vi "isDone.vi"(8 "error in (no error)":errorcluster, 11 "ChirpWave in":refnum<class "ChirpWave.lvclass">) -> (0 "error out":errorcluster, 2 "isDone?":bool=TRUE, 3 "ChirpWave out":refnum<class "ChirpWave.lvclass">)   [LabVIEW 2015, in "ChirpWave.lvclass"]
uses:
  ChirpWave.lvclass
  ChirpWave.lvclass/ChirpWave.ctl
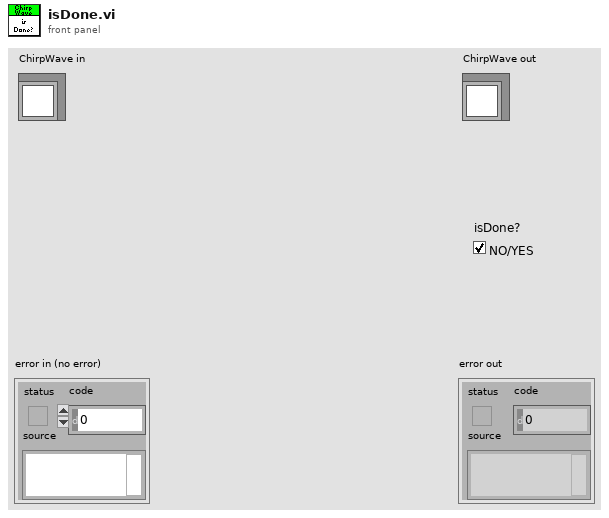
[diagram p1: front panel]
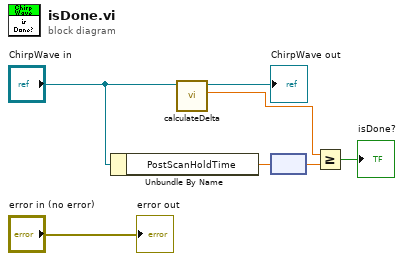
[diagram p0: block diagram]
diagram:
  n1 = Unbundle By Name("ChirpWave in") -> ("PostScanHoldTime"=w2:dbl[unit])
  n2 = call "calculateDelta.vi"("ChirpWave in"="ChirpWave in") -> ("Delta Timestamp"=w5:dbl, "ChirpWave out"=→"ChirpWave out":refnum<class "ChirpWave.lvclass">)  [unwired: 8 in, 1 out]
  n3 = node(w2) -> (w3:dbl)
  n4 = Greater Or Equal?(x=w5, y=w3) -> (x >= y?=→"isDone?":bool)
  "error out" <- "error in (no error)"
